vi "ScanNetwork_Example.vi"(8 "Fehler (Eingang, kein Fehler)":errorcluster) -> (0 "Fehler (Ausgang)":errorcluster, 2 "NetworkDevices Array":string[][](array[string]))   [LabVIEW 2016]
panel:
  in  "Network Devices":i32(listbox)=-1
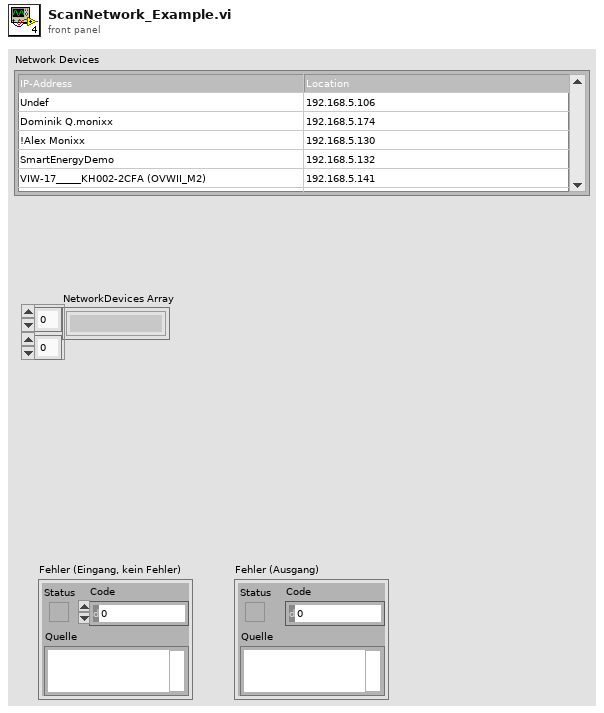
[diagram p1: front panel]
types:
  T1 = enum16{"Bool", "Snippet", "Struct", "Int64", "Int32", "Float", "Double", "String"}
  T2 = typedef "girpcutil_params.ctl" = cluster{"ConnectionHandle":i32, "DLL-Handle":cluster{"DLL Path":path, "Is32Bit":bool}}
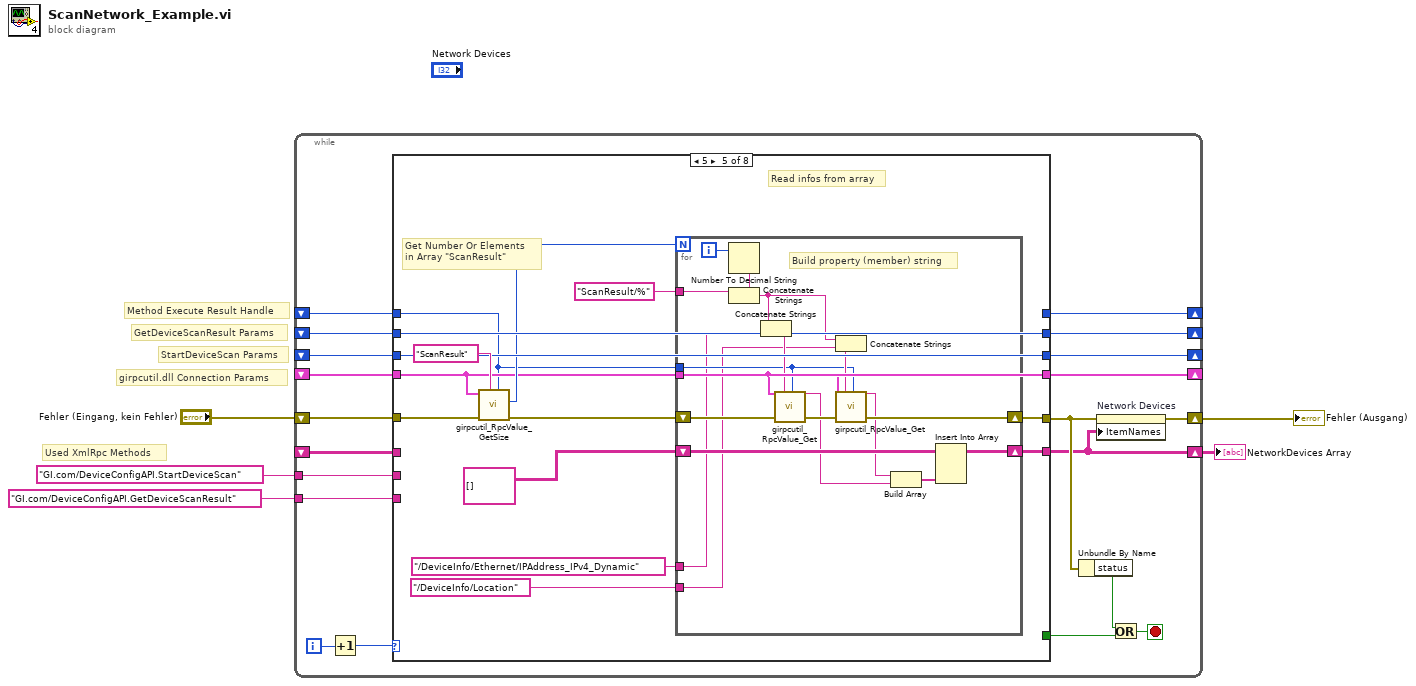
[diagram p0: block diagram]
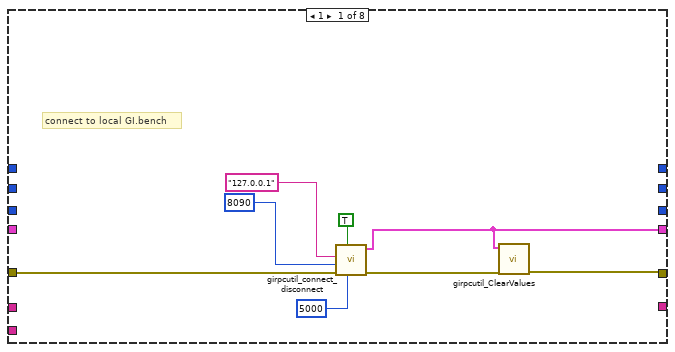
[diagram p2: hidden frame]
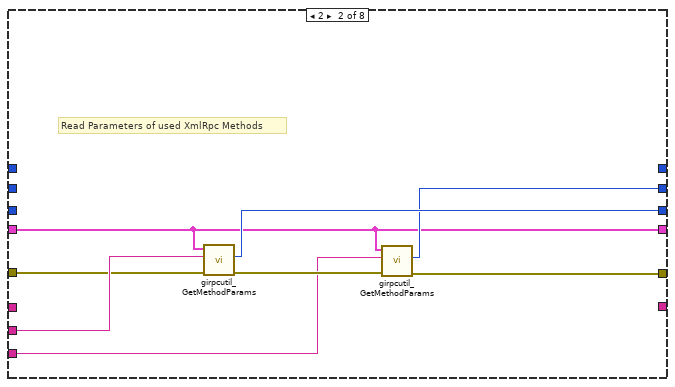
[diagram p3: hidden frame]
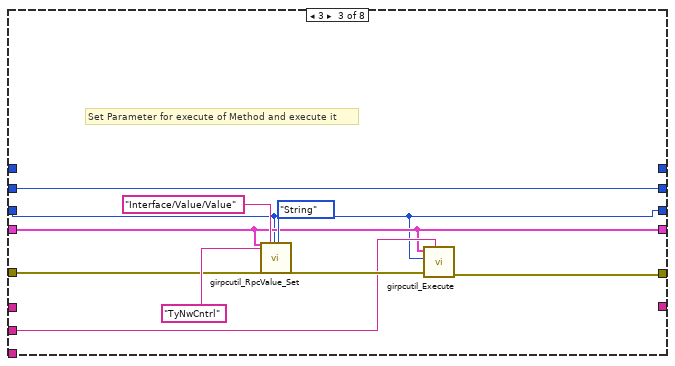
[diagram p4: hidden frame]
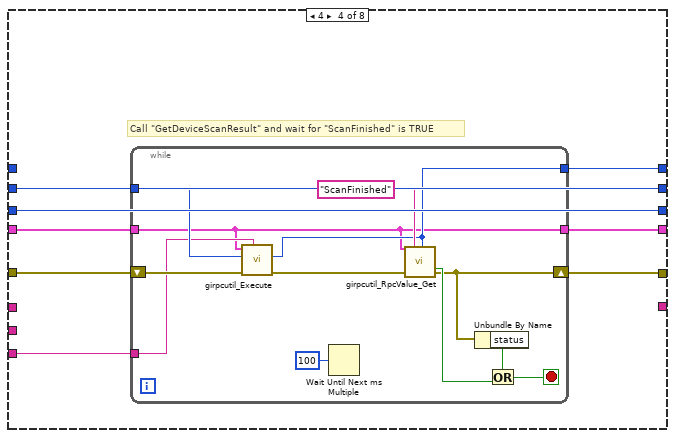
[diagram p5: hidden frame]
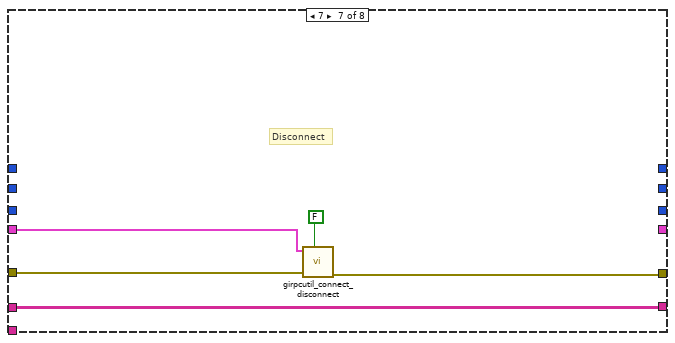
[diagram p7: hidden frame]
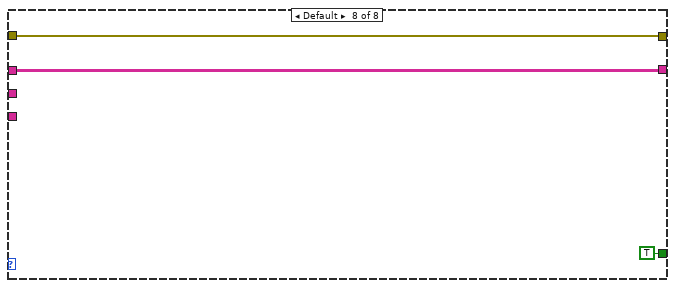
[diagram p8: hidden frame]
diagram:
  # "Method Execute Result Handle"
  # "girpcutil.dll Connection Params"
  # "Used XmlRpc Methods"
  # "GetDeviceScanResult Params"
  # "StartDeviceScan Params"
  n1 = while {
    shift-right: [w22] -> _
    shift-left: _ -> [w16]
    tunnel: "GI.com/DeviceConfigAPI.StartDeviceScan" ("methodName") -> [w21]
    tunnel: "GI.com/DeviceConfigAPI.GetDeviceScanResult" ("methodName") -> [w20]
    shift-right: [w8] -> w2
    shift-left: "Fehler (Eingang, kein Fehler)" -> [w23]
    shift-right: [w15] -> _
    shift-left: _ -> [w14]
    shift-right: [w13] -> _
    shift-left: _ -> [w12]
    shift-right: [w11] -> _
    shift-left: _ -> [w10]
    shift-right: [w7] -> w1
    shift-left: _ -> [w6]
    i -> [w25]
    stop <- w19 stop-if-true
    n2 = Increment(x=w25) -> (x+1=w24:i32)
    n3 = case shown="5" w24 {
      tunnel: [_ _ _ _ _ _ _ TRUE] -> w18
      tunnel: w23 -> [w29 w38 w46 w59 w85 w105 w109 w112]
      tunnel: [w26 w34 w43 w53 w79 _ _ _] -> w22
      tunnel: w21 -> [_ w40 w47 _ _ _ _ _]
      tunnel: w20 -> [_ w39 _ w57 _ _ _ _]
      tunnel: [w27 w37 w45 w56 w77 w105 w108 w112] -> w9
      tunnel: w16 -> [_ w34 w43 w58 w79 _ w107 _]
      tunnel: [_ w36 w42 w54 w82 _ _ _] -> w15
      tunnel: w14 -> [_ _ w42 w54 w82 _ _ _]
      tunnel: [_ w35 w44 w52 w83 _ _ _] -> w13
      tunnel: w12 -> [_ _ w44 w52 w83 _ _ _]
      tunnel: [_ _ _ w55 _ _ _ _] -> w11
      tunnel: w10 -> [_ _ _ _ w78 _ _ _]
      tunnel: [_ _ _ _ w75 w104 w106 w111] -> w7
      tunnel: w6 -> [_ _ _ _ _ w104 w106 w111]
      frame 1 {
        # "connect to local GI.bench"
        n4 = call "girpcutil_connect_disconnect.vi"("timeout"=u32 5000, "Connect"=TRUE, "Fehler (Eingang, kein Fehler)"=w29, "port"=u32 8090, "host"="127.0.0.1") -> ("Fehler (Ausgang)"=w28:errorcluster, "girpcutil_params 2"=w26:T2)  [unwired: 5 in]
        n5 = call "girpcutil_ClearValues.vi"("Fehler (Eingang, kein Fehler)"=w28, "girpcutil_params"=w26) -> ("error IO"=w27:errorcluster)  [unwired: 9 in]
      }
      frame 2 {
        # "Read Parameters of used XmlRpc Methods"
        n6 = call "girpcutil_GetMethodParams.vi"("Fehler (Eingang, kein Fehler)"=w38, "methodName"=w40, "girpcutil_params"=w34) -> ("Fehler (Ausgang)"=w41:errorcluster, "param handle out"=w36:i32)  [unwired: 7 in]
        n7 = call "girpcutil_GetMethodParams.vi"("Fehler (Eingang, kein Fehler)"=w41, "methodName"=w39, "girpcutil_params"=w34) -> ("Fehler (Ausgang)"=w37:errorcluster, "param handle out"=w35:i32)  [unwired: 7 in]
      }
      frame 3 {
        # "Set Parameter for execute of Method and execute it"
        n8 = call "girpcutil_RpcValue_Set.vi"("girpcutil_params"=w43, "StringValue or Snippet"="TyNwCntrl", "Fehler (Eingang, kein Fehler)"=w46, "MemberName"="Interface/Value/Value", "param handle"=w42, "DataType"=T1."String") -> ("Fehler (Ausgang)"=w48:errorcluster)  [unwired: 21 in]
        n9 = call "girpcutil_Execute.vi"("methodName"=w47, "Fehler (Eingang, kein Fehler)"=w48, "params"=w42, "girpcutil_params"=w43) -> ("Fehler (Ausgang)"=w45:errorcluster)  [unwired: 6 in, 1 out]
      }
      frame 4 {
        # "Call \"GetDeviceScanResult\" and wait for \"ScanFinished\" is TRUE"
        n10 = while {
          tunnel: w52 -> [w70]
          tunnel: w58 -> [w60]
          shift-right: [w64] -> w56
          shift-left: w59 -> [w71]
          tunnel: w57 -> [w61]
          tunnel: [w62] -> w55
          tunnel: [w60] -> w53
          stop <- w67 stop-if-true
          n11 = call "girpcutil_Execute.vi"("methodName"=w61, "Fehler (Eingang, kein Fehler)"=w71, "params"=w70, "girpcutil_params"=w60) -> ("Fehler (Ausgang)"=w69:errorcluster, "results"=w62:i32)  [unwired: 6 in]
          n12 = Wait Until Next ms Multiple(millisecond multiple=u32 100) -> ()  [unwired: 1 out]
          n13 = call "girpcutil_RpcValue_Get.vi"("girpcutil_params"=w60, "Fehler (Eingang, kein Fehler)"=w69, "member"="ScanFinished", "value"=w62) -> ("BoolResult"=w66:bool, "Fehler (Ausgang)"=w64:errorcluster)  [unwired: 19 in, 3 out]
          n14 = Unbundle By Name(w64) -> ("status"=w63:bool)
          n15 = Or(x=w63, y=w66) -> (x .or. y?=w67:bool)
        }
      }
      frame 5 {
        # "Read infos from array"
        # "Get Number Or Elements \nin Array \"ScanResult\""
        n16 = call "girpcutil_RpcValue_GetSize.vi"("param handle"=w78, "member"="ScanResult", "Fehler (Eingang, kein Fehler)"=w85, "girpcutil_params"=w79) -> ("Fehler (Ausgang)"=w80:errorcluster, "size"=w81:u64)  [unwired: 6 in]
        n17 = for {
          N: w81 -> [_]
          tunnel: w79 -> [w94]
          tunnel: w78 -> [w95]
          shift-right: [w102] -> w77
          shift-left: w80 -> [w98]
          shift-right: [w92] -> w75
          shift-left: string[][] [] -> [w93]
          tunnel: "/DeviceInfo/Ethernet/IPAddress_IPv4_Dynamic" ("string") -> [w88]
          tunnel: "/DeviceInfo/Location" ("string") -> [w87]
          tunnel: "ScanResult/%" ("string") -> [w86]
          i -> [w101]
          # "Build property (member) string"
          n18 = Number To Decimal String(number=w101) -> (decimal integer string=w103:string)  [unwired: 1 in]
          n19 = Concatenate Strings(w86, w103) -> (w99:string)
          n20 = Concatenate Strings(w99, w88) -> (w96:string)
          n21 = call "girpcutil_RpcValue_Get.vi"("girpcutil_params"=w94, "Fehler (Eingang, kein Fehler)"=w98, "member"=w96, "value"=w95) -> ("StringResult"=w89:string, "Fehler (Ausgang)"=w97:errorcluster)  [unwired: 19 in, 3 out]
          n22 = Concatenate Strings(w99, w87) -> (w100:string)
          n23 = call "girpcutil_RpcValue_Get.vi"("girpcutil_params"=w94, "Fehler (Eingang, kein Fehler)"=w97, "member"=w100, "value"=w95) -> ("StringResult"=w90:string, "Fehler (Ausgang)"=w102:errorcluster)  [unwired: 19 in, 3 out]
          n24 = Build Array(w90, w89) -> (w91:string[])
          n25 = Insert Into Array(array=w93, new element=w91) -> (w92:string[][])  [unwired: 2 in]
        }
      }
      frame 6 {
      }
      frame 7 {
        # "Disconnect"
        n26 = call "girpcutil_connect_disconnect.vi"("Connect"=FALSE, "Fehler (Eingang, kein Fehler)"=w109, "girpcutil_params"=w107) -> ("Fehler (Ausgang)"=w108:errorcluster)  [unwired: 7 in, 1 out]
      }
      frame Default {
      }
    }
    n27 = Unbundle By Name(w9) -> ("status"=w17:bool)
    n28 = property on="Network Devices" class="MCListbox (strict)"(error in=w9, "ItemNames"=w7) -> (error out=w8:errorcluster)  [unwired: 1 in, 1 out]
    n29 = Or(x=w17, y=w18) -> (x .or. y?=w19:bool)
  }
  "Fehler (Ausgang)" <- w2
  "NetworkDevices Array" <- w1
